vi "Calcu_STD Pressure_PB.vi"(6 "Resolution":string[][](array[string]), 9 "Dead Weight":string[][](array[string]), 10 "Cal STD":string[](array[string]), 11 "Condition":string[][](array[string])) -> (0 "배열":dbl[](array[numeric]), 1 "Mass set":string[][](array[string]), 2 "Uncertainty":string[][](array[string]), 3 "Data Out":string[][](array[string]), 4 "Weight set":string[][](array[string]), 5 "STD Data":string[][](array[string]))   [LabVIEW 2020]
uses:
  Controls/Cmd_File path.ctl
  Controls/Cmd_File Type.ctl
  Public/Polymorph/Data Class_2D Str.vi
  Variables/Global_Cal Info.vi
  Public/Polymorph/Array Dedup_2D Str.vi
  Public/Polymorph/Sort_2D Str.vi
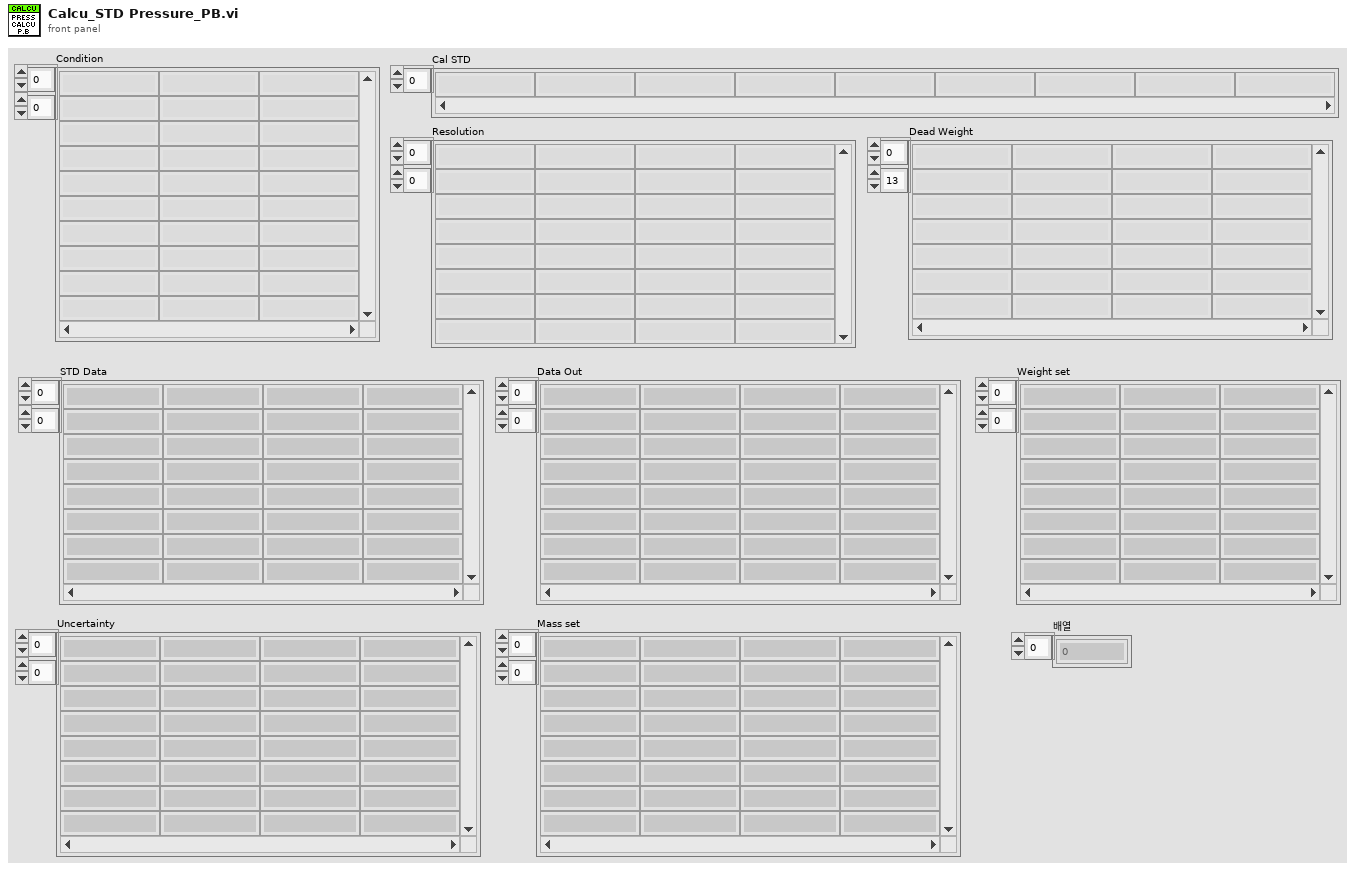
[diagram p1: front panel]
types:
  T1 = typedef "Cmd_File Type.ctl" = enum16{"엑셀", "엑셀(2003)", "텍스트", "설정", "2진", "VI", "CSV", "LOG", "폴더"}
  T2 = typedef "Cmd_File path.ctl" = enum16{"에러로그", "데이터파일경로", "성적서원본", "지난성적서", "Data Files", "경로생성", "Updater", "Template", "설정파일경로", "FTP Upload", "Update 경로", "어플리케이션"}
  T3 = cluster{"세부분류코드":string, "형식":string, "옵션":string, "측정기명":string, "EXCEL파일명":string, "TEMP":string}
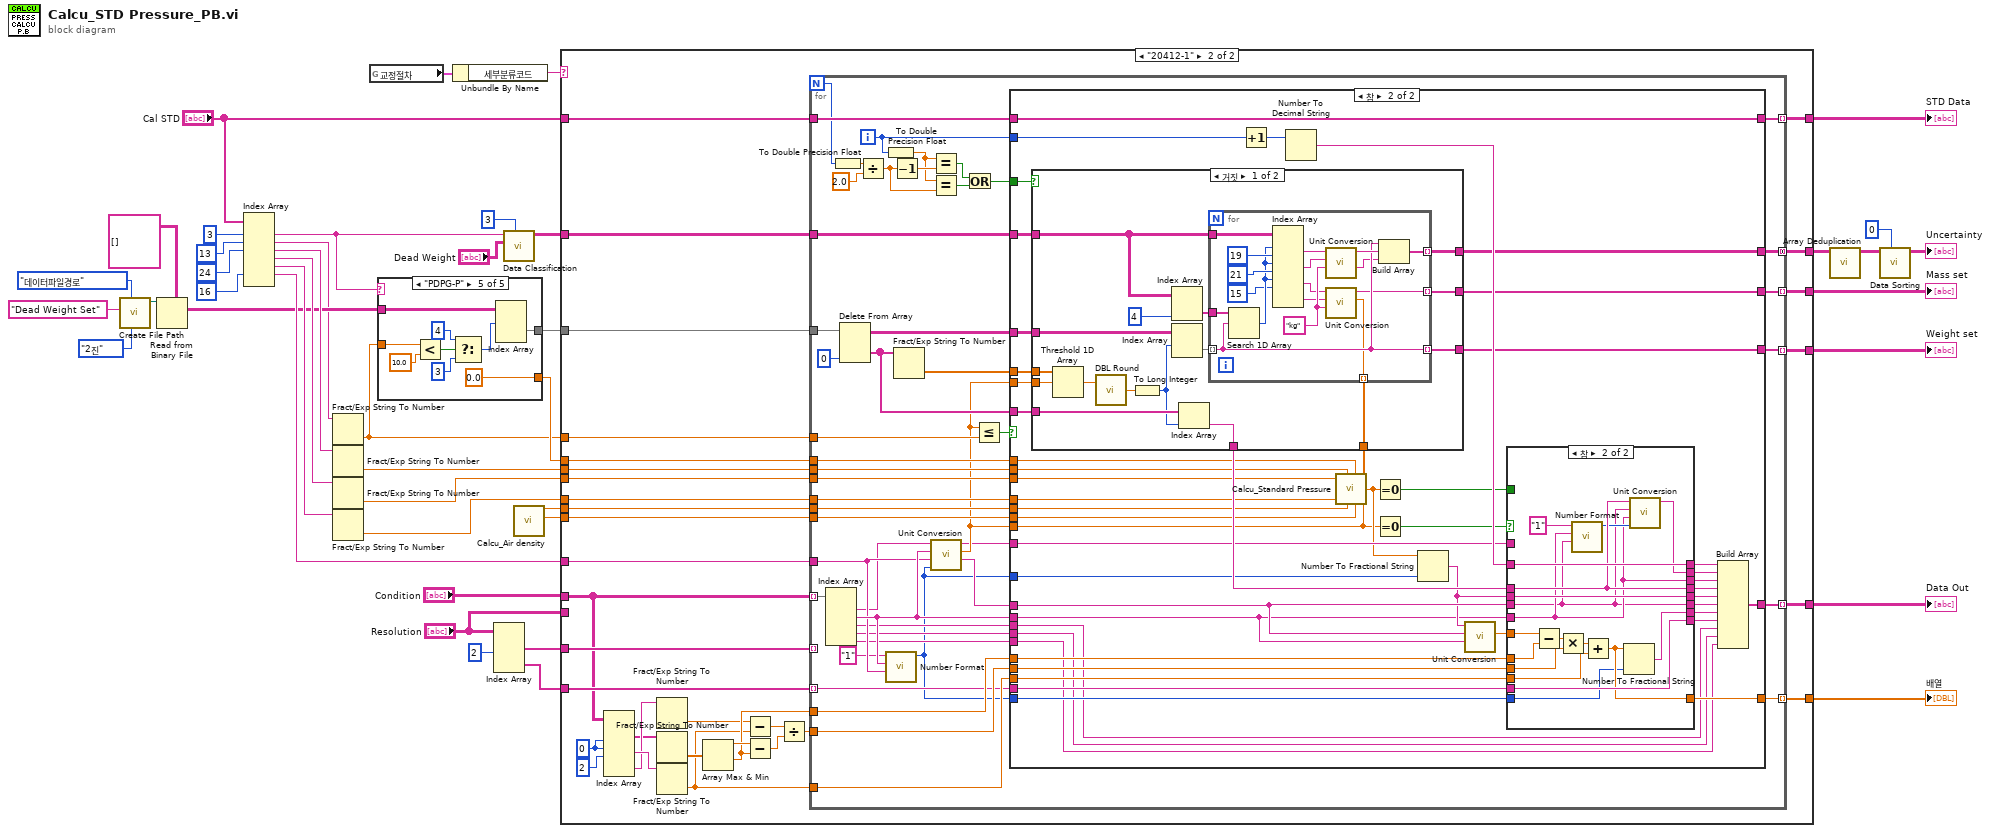
[diagram p0: block diagram]
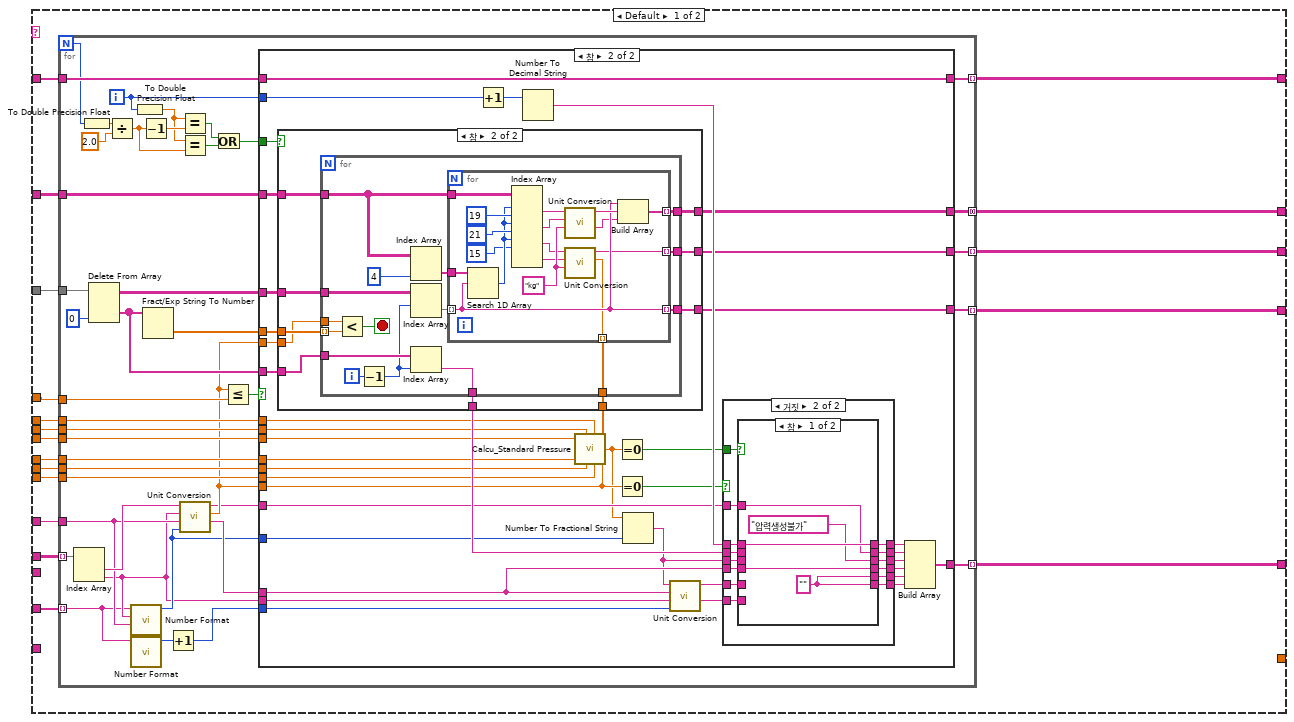
[diagram p2: hidden frame]
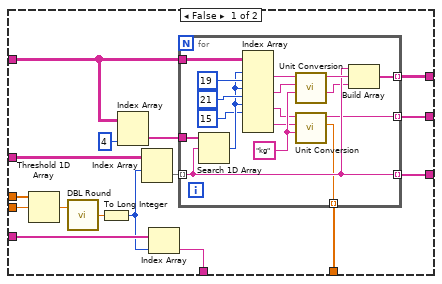
[diagram p6: hidden frame]
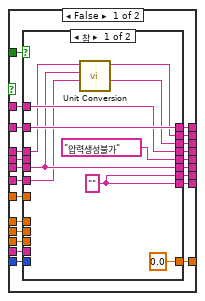
[diagram p8: hidden frame]
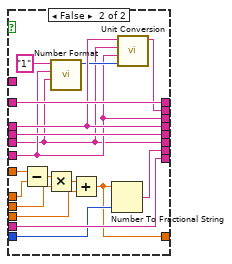
[diagram p9: hidden frame]
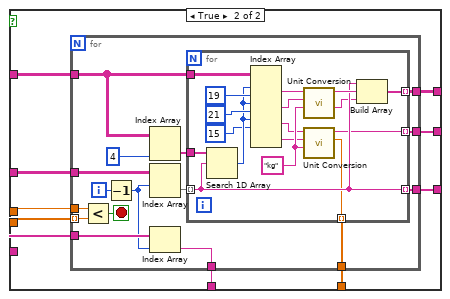
[diagram p10: hidden frame]
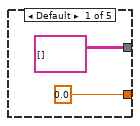
[diagram p11: hidden frame]
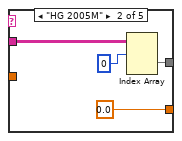
[diagram p12: hidden frame]
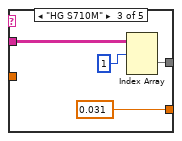
[diagram p13: hidden frame]
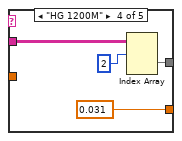
[diagram p14: hidden frame]
diagram:
  n1 = call "Create File Path.vi"("파일타입"=Cmd_File_Type."2진", "항목"=Cmd_File_path."데이터파일경로", "문자열 in"="Dead Weight Set") -> ("파일경로"=w7:path)  [unwired: 5 in, 3 out]
  n2 = Read from Binary File(5:string[][][] [], 11:w7) -> (2:w11:string[][][])  [unwired: 4 in, 3 out]
  n3 = Index Array(array="Cal STD", index #1=3 ("인덱스"), index #2=13 ("인덱스"), index #3=24 ("인덱스"), index #6=16 ("인덱스")) -> (element #1=w17:string, element #2=w6:string, element #3=w21:string, element #4=w20:string, element #5=w19:string, element #6=w14:string)  [unwired: 3 in, 1 out]
  n4 = Fract/Exp String To Number(string=w6) -> (number=w5:dbl)  [unwired: 3 in, 1 out]
  n5 = Fract/Exp String To Number(string=w21) -> (number=w35:dbl)  [unwired: 3 in, 1 out]
  n6 = Fract/Exp String To Number(string=w20) -> (number=w37:dbl)  [unwired: 3 in, 1 out]
  n7 = Fract/Exp String To Number(string=w19) -> (number=w36:dbl)  [unwired: 3 in, 1 out]
  n8 = global read "Global_Cal Info.vi" "교정절차"() -> (w24:T3)
  n9 = case shown="\"PDPG-P\"" w17 {
    tunnel: [string[][] [] ("테이블 컨트롤 2") w48 w51 w55 w65] -> w43
    tunnel: [0.0 0.0 0.031 0.031 0.0] -> w38
    tunnel: w11 -> [_ w49 w53 w57 w66]
    tunnel: w5 -> [_ _ _ _ w64]
    frame Default {
    }
    frame "HG 2005M" {
      n10 = Index Array(array=w49, index (dim 0)=0 ("인덱스 (페이지)")) -> (element=w48:string[][])  [unwired: 2 in]
    }
    frame "HG S710M" {
      n11 = Index Array(array=w53, index (dim 0)=1 ("인덱스 (페이지)")) -> (element=w51:string[][])  [unwired: 2 in]
    }
    frame "HG 1200M" {
      n12 = Index Array(array=w57, index (dim 0)=2 ("인덱스 (페이지)")) -> (element=w55:string[][])  [unwired: 2 in]
    }
    frame "PDPG-P" {
      n13 = Less?(x=w64, y=10.0) -> (x < y?=w62:bool)
      n14 = Select(t=4 ("인덱스 (페이지)"), s=w62, f=3 ("인덱스 (페이지)")) -> (s? t:f=w60:i32)
      n15 = Index Array(array=w66, index (dim 0)=w60) -> (element=w65:string[][])  [unwired: 2 in]
    }
  }
  n16 = Unbundle By Name(w24) -> ("세부분류코드"=w2:string)
  n17 = Index Array(array="Resolution", index (col) #1=2 ("비활성화된 인덱스 (열)")) -> (element #1=w33:string[], element #2=w23:string[])  [unwired: 3 in]
  n18 = call-poly "Data Classification.vi"("인덱스"=3, "DATA 입력"="Dead Weight", "검색 문자열"=w17) -> ("DATA 출력"=w40:string[][])  [unwired: 4 in, 4 out]
  n19 = call "Calcu_Air density.vi"() -> ("t(℃)"=w4:dbl, "ρ_air"=w39:dbl)  [unwired: 10 in]
  n20 = case shown="\"20412-1\"" w2 {
    tunnel: [w85 w306] -> w44
    tunnel: "Condition" -> [w84 w278]
    tunnel: w14 -> [w83 w305]
    tunnel: w43 -> [w82 w304]
    tunnel: w40 -> [w81 w303]
    tunnel: w39 -> [w80 w302]
    tunnel: w38 -> [w79 w301]
    tunnel: w37 -> [w78 w300]
    tunnel: w4 -> [w77 w299]
    tunnel: w36 -> [w76 w298]
    tunnel: w35 -> [w75 w297]
    tunnel: w5 -> [w74 w296]
    tunnel: w33 -> [w73 w295]
    tunnel: [w72 w294] -> w32
    tunnel: "Cal STD" -> [w71 w293]
    tunnel: [w70 w292] -> w27
    tunnel: [w69 w291] -> w26
    tunnel: [w68 w290] -> w25
    tunnel: w23 -> [_ w289]
    tunnel: [_ w288] -> w13
    tunnel: "Resolution" -> [_ _]
    frame Default {
      n21 = for {
        N -> [w101]
        tunnel: [w126] -> w85 mode=indexing
        tunnel: w84 -> [w125] mode=indexing
        tunnel: w83 -> [w104]
        tunnel: w82 -> [w122]
        tunnel: [w118] -> w69 mode=indexing
        tunnel: w81 -> [w121]
        tunnel: w80 -> [w117]
        tunnel: w79 -> [w116]
        tunnel: w75 -> [w115]
        tunnel: w78 -> [w114]
        tunnel: w77 -> [w113]
        tunnel: w76 -> [w112]
        tunnel: w74 -> [w110]
        tunnel: w73 -> [w88] mode=indexing
        tunnel: [w108] -> w72 mode=concatenating
        tunnel: w71 -> [w107]
        tunnel: [w106] -> w70 mode=indexing
        tunnel: [w105] -> w68 mode=indexing
        i -> [w97]
        n22 = Index Array(array=w125) -> (element #1=w124:string, element #2=w89:string)  [unwired: 2 in]
        n23 = To Double Precision Float(number=w101) -> (double precision float=w95:dbl)
        n24 = Delete From Array(array=w122, index (col)=0 ("비활성화된 인덱스 (열)")) -> (deleted portion=w103:string[], array with subset deleted=w119:string[][])  [unwired: 2 in]
        n25 = Divide(x=w95, y=2.0) -> (x/y=w99:dbl)
        n26 = call "Number Format.vi"("기준단위"=w104, "입력단위"=w89, "입력값"=w88) -> ("정밀도(단위적용)"=w91:i32)  [unwired: 8 in]
        n27 = call "Number Format.vi"("입력값"=w88) -> ("정밀도(단위적용)"=w87:i32)  [unwired: 10 in]
        n28 = To Double Precision Float(number=w97) -> (double precision float=w96:dbl)
        n29 = Decrement(x=w99) -> (x-1=w98:dbl)
        n30 = Fract/Exp String To Number(string=w103) -> (number=w123:dbl[])  [unwired: 3 in, 1 out]
        n31 = Increment(x=w87) -> (x+1=w86:i32)
        n32 = Equal?(x=w96, y=w98) -> (x = y?=w94:bool)
        n33 = Equal?(x=w96, y=w99) -> (x = y?=w93:bool)
        n34 = call "Unit Conversion.vi"("소수점 자리수"=w91, "환산단위"=w104, "입력단위"=w89, "입력값"=w124) -> ("환산단위"=w111:string, "환산값 (DBL)"=w102:dbl, "환산값 (string)"=w92:string)  [unwired: 2 in, 3 out]
        n35 = Or(x=w94, y=w93) -> (x .or. y?=w90:bool)
        n36 = Less Or Equal?(x=w102, y=w110) -> (x <= y?=w109:bool)
        n37 = case shown="참" w109 {
          tunnel: w97 -> [_ w166]
          tunnel: [_ w145] -> w126
          tunnel: w123 -> [_ w158]
          tunnel: w121 -> [_ w163]
          tunnel: w119 -> [_ w156]
          tunnel: [_ w137] -> w118
          tunnel: w117 -> [_ w130]
          tunnel: w116 -> [_ w134]
          tunnel: w115 -> [_ w133]
          tunnel: w114 -> [_ w132]
          tunnel: w102 -> [_ w157]
          tunnel: w113 -> [_ w129]
          tunnel: w112 -> [_ w131]
          tunnel: w111 -> [_ w149]
          tunnel: w89 -> [_ w150]
          tunnel: [_ w162] -> w108
          tunnel: w107 -> [_ w161]
          tunnel: [_ w161] -> w106
          tunnel: [_ w138] -> w105
          tunnel: w91 -> [_ w152]
          tunnel: w103 -> [_ w160]
          tunnel: w102 -> [_ w128]
          tunnel: w90 -> [_ w155]
          tunnel: w92 -> [_ w153]
          tunnel: w86 -> [_ w136]
          frame False {
          }
          frame True {
            n38 = case shown="참" w155 {
              tunnel: w163 -> [w209 w240]
              tunnel: [w206 w239] -> w137
              tunnel: [w207 w238] -> w162
              tunnel: [w204 w237] -> w135
              tunnel: [w205 w236] -> w138
              tunnel: w160 -> [w211 w235]
              tunnel: [w208 w234] -> w159
              tunnel: w158 -> [w202 w233]
              tunnel: w157 -> [w201 w232]
              tunnel: w156 -> [w210 w231]
              frame False {
                n39 = Threshold 1D Array(2:w201, 3:w202) -> (0:w198:dbl)  [unwired: 1 in]
                n40 = call "DBL Round.vi"("DBL in"=w198) -> ("DBL out"=w199:dbl)  [unwired: 2 in]
                n41 = To Long Integer(number=w199) -> (32bit integer=w203:i32)
                n42 = Index Array(array=w209, index (col)=4 ("비활성화된 인덱스 (열)")) -> (element=w213:string[])  [unwired: 1 in]
                n43 = Index Array(array=w210, index (row)=w203) -> (element=w212:string[])  [unwired: 1 in]
                n44 = Index Array(array=w211, index=w203) -> (element=w208:string)
                n45 = for {
                  tunnel: w212 -> [w223] mode=indexing
                  tunnel: w209 -> [w230]
                  tunnel: [w221] -> w206 mode=indexing
                  tunnel: [w224] -> w207 mode=indexing
                  tunnel: [w220] -> w204 mode=indexing
                  tunnel: [w223] -> w205 mode=indexing
                  tunnel: w213 -> [w219]
                  w222 = "kg" ("환산단위")
                  n46 = Search 1D Array(1D array=w219, element=w223) -> (index of element=w217:i32)  [unwired: 1 in]
                  n47 = Index Array(array=w230, index (row) #1=w217, index (col) #1=19 ("인덱스 (열)"), index (row) #2=w217, index (col) #2=21 ("인덱스 (열)"), index (row) #3=w217, index (col) #3=15 ("비활성화된 인덱스 (열)")) -> (element #1=w227:string, element #2=w226:string, element #3=w215:string, element #4=w214:string)  [unwired: 2 in]
                  n48 = call "Unit Conversion.vi"("환산단위"=w222, "입력단위"=w226, "입력값"=w227) -> ("환산단위"=w218:string, "환산값 (string)"=w225:string)  [unwired: 3 in, 4 out]
                  n49 = call "Unit Conversion.vi"("환산단위"=w222, "입력단위"=w214, "입력값"=w215) -> ("환산값 (DBL)"=w220:dbl, "환산값 (string)"=w221:string)  [unwired: 3 in, 4 out]
                  n50 = Build Array(w223, w225, w218) -> (w224:string[])
                }
              }
              frame True {
                n51 = for {
                  tunnel: w232 -> [w255]
                  tunnel: w233 -> [w256] mode=indexing
                  tunnel: w231 -> [w253]
                  tunnel: [w250] -> w239
                  tunnel: w240 -> [w242]
                  tunnel: [w249] -> w238
                  tunnel: [w248] -> w237
                  tunnel: [w247] -> w236
                  tunnel: w235 -> [w246]
                  tunnel: [w244] -> w234
                  i -> [w252]
                  stop <- w254 stop-if-true
                  n52 = Less?(x=w255, y=w256) -> (x < y?=w254:bool)
                  n53 = Decrement(x=w252) -> (x-1=w245:i32)
                  n54 = Index Array(array=w242, index (col)=4 ("비활성화된 인덱스 (열)")) -> (element=w241:string[])  [unwired: 1 in]
                  n55 = Index Array(array=w253, index (row)=w245) -> (element=w251:string[])  [unwired: 1 in]
                  n56 = Index Array(array=w246, index=w245) -> (element=w244:string)
                  n57 = for {
                    tunnel: w251 -> [w266] mode=indexing
                    tunnel: w242 -> [w273]
                    tunnel: [w264] -> w250 mode=indexing
                    tunnel: [w267] -> w249 mode=indexing
                    tunnel: [w263] -> w248 mode=indexing
                    tunnel: [w266] -> w247 mode=indexing
                    tunnel: w241 -> [w262]
                    w265 = "kg" ("환산단위")
                    n58 = Search 1D Array(1D array=w262, element=w266) -> (index of element=w260:i32)  [unwired: 1 in]
                    n59 = Index Array(array=w273, index (row) #1=w260, index (col) #1=19 ("인덱스 (열)"), index (row) #2=w260, index (col) #2=21 ("인덱스 (열)"), index (row) #3=w260, index (col) #3=15 ("비활성화된 인덱스 (열)")) -> (element #1=w270:string, element #2=w269:string, element #3=w258:string, element #4=w257:string)  [unwired: 2 in]
                    n60 = call "Unit Conversion.vi"("환산단위"=w265, "입력단위"=w269, "입력값"=w270) -> ("환산단위"=w261:string, "환산값 (string)"=w268:string)  [unwired: 3 in, 4 out]
                    n61 = call "Unit Conversion.vi"("환산단위"=w265, "입력단위"=w257, "입력값"=w258) -> ("환산값 (DBL)"=w263:dbl, "환산값 (string)"=w264:string)  [unwired: 3 in, 4 out]
                    n62 = Build Array(w266, w268, w261) -> (w267:string[])
                  }
                }
              }
            }
            n63 = Increment(x=w166) -> (x+1=w165:i32)
            n64 = Number To Decimal String(number=w165) -> (decimal integer string=w164:string)  [unwired: 1 in]
            n65 = call "Calcu_Standard Pressure.vi"("λ"=w132, "A0"=w133, "Ts"=w131, "ρa"=w130, "σ"=w134, "M"=w135, "Ta"=w129, "P"=w128) -> ("결과"=w127:dbl)  [unwired: 1 in]
            n66 = Equal To 0?(x=w127) -> (x = 0?=w151:bool)
            n67 = Equal To 0?(x=w128) -> (x = 0?=w154:bool)
            n68 = Number To Fractional String(number=w127, precision (6)=w152) -> (F-format string=w148:string)  [unwired: 2 in]
            n69 = call "Unit Conversion.vi"("소수점 자리수"=w136, "환산단위"=w150, "입력단위"=w149, "입력값"=w148) -> ("환산단위"=w146:string, "환산값 (string)"=w147:string)  [unwired: 2 in, 4 out]
            n70 = case shown="거짓" w154 {
              tunnel: w164 -> [w172 w186]
              tunnel: w149 -> [w169 w185]
              tunnel: w159 -> [w171 w184]
              tunnel: w153 -> [_ w183]
              tunnel: w148 -> [w170 w182]
              tunnel: w151 -> [_ w181]
              tunnel: w147 -> [w168 w179]
              tunnel: w146 -> [w167 w180]
              tunnel: [w172 w178] -> w144
              tunnel: [w171 w177] -> w143
              tunnel: [w170 w176] -> w142
              tunnel: [w169 w175] -> w141
              tunnel: [w168 w174] -> w140
              tunnel: [w167 w173] -> w139
              frame True {
              }
              frame False {
                n71 = case shown="참" w181 {
                  tunnel: w186 -> [w191 w197]
                  tunnel: w185 -> [w188 w194]
                  tunnel: w184 -> [_ w196]
                  tunnel: w183 -> [w190 _]
                  tunnel: w182 -> [_ w195]
                  tunnel: w180 -> [_ w192]
                  tunnel: w179 -> [_ w193]
                  tunnel: [w191 w197] -> w178
                  tunnel: [w190 w196] -> w177
                  tunnel: ["압력생성불가" w195] -> w176
                  tunnel: [w188 w194] -> w175
                  tunnel: [w187 w193] -> w174
                  tunnel: [w187 w192] -> w173
                  frame True {
                    w187 = ""
                  }
                  frame False {
                  }
                }
              }
            }
            n72 = Build Array(w144, w143, w142, w141, w140, w139) -> (w145:string[])
          }
        }
      }
    }
    frame "20412-1" {
      w275 = 0 ("비활성화된 인덱스 (열)")
      n73 = Index Array(array=w278, index (col) #1=w275, index (row) #2=w275, index (col) #2=2 ("인덱스 (행)")) -> (element #1=w274:string[], element #2=w277:string, element #3=w276:string)  [unwired: 3 in]
      n74 = Fract/Exp String To Number(string=w276) -> (number=w281:dbl)  [unwired: 3 in, 1 out]
      n75 = Fract/Exp String To Number(string=w274) -> (number=w282:dbl[])  [unwired: 3 in, 1 out]
      n76 = Fract/Exp String To Number(string=w277) -> (number=w280:dbl)  [unwired: 3 in, 1 out]
      n77 = Array Max & Min(array=w282) -> (max value=w284:dbl, min value=w283:dbl)  [unwired: 2 out]
      n78 = Subtract(x=w281, y=w280) -> (x-y=w286:dbl)
      n79 = Subtract(x=w284, y=w283) -> (x-y=w285:dbl)
      n80 = Divide(x=w286, y=w285) -> (x/y=w287:dbl)
      n81 = for {
        N -> [w328]
        tunnel: [w353] -> w306 mode=indexing
        tunnel: w278 -> [w352] mode=indexing
        tunnel: w305 -> [w331]
        tunnel: w304 -> [w350]
        tunnel: [w346] -> w291 mode=indexing
        tunnel: w303 -> [w349]
        tunnel: w302 -> [w345]
        tunnel: w301 -> [w344]
        tunnel: w297 -> [w343]
        tunnel: w300 -> [w342]
        tunnel: w299 -> [w341]
        tunnel: w298 -> [w340]
        tunnel: w296 -> [w338]
        tunnel: w295 -> [_] mode=indexing
        tunnel: [w336] -> w294 mode=concatenating
        tunnel: w293 -> [w335]
        tunnel: [w334] -> w292 mode=indexing
        tunnel: [w333] -> w290 mode=indexing
        tunnel: w287 -> [w317]
        tunnel: w283 -> [w316]
        tunnel: w280 -> [w315]
        tunnel: w289 -> [w314] mode=indexing
        tunnel: [w313] -> w288 mode=indexing
        i -> [w324]
        n82 = Index Array(array=w352) -> (element #1=w308:string, element #2=w332:string, element #3=w312:string, element #4=w311:string, element #5=w310:string)  [unwired: 5 in]
        n83 = To Double Precision Float(number=w328) -> (double precision float=w322:dbl)
        n84 = Delete From Array(array=w350, index (col)=0 ("비활성화된 인덱스 (열)")) -> (deleted portion=w330:string[], array with subset deleted=w347:string[][])  [unwired: 2 in]
        n85 = Divide(x=w322, y=2.0) -> (x/y=w326:dbl)
        n86 = To Double Precision Float(number=w324) -> (double precision float=w323:dbl)
        n87 = call "Number Format.vi"("기준단위"=w331, "입력단위"=w332, "입력값"="1") -> ("정밀도(단위적용)"=w309:i32)  [unwired: 8 in]
        n88 = Decrement(x=w326) -> (x-1=w325:dbl)
        n89 = Fract/Exp String To Number(string=w330) -> (number=w351:dbl[])  [unwired: 3 in, 1 out]
        n90 = Equal?(x=w323, y=w325) -> (x = y?=w321:bool)
        n91 = Equal?(x=w323, y=w326) -> (x = y?=w320:bool)
        n92 = call "Unit Conversion.vi"("소수점 자리수"=w309, "환산단위"=w331, "입력단위"=w332, "입력값"=w308) -> ("환산단위"=w339:string, "환산값 (DBL)"=w329:dbl, "환산값 (string)"=w318:string)  [unwired: 2 in, 3 out]
        n93 = Or(x=w321, y=w320) -> (x .or. y?=w319:bool)
        n94 = Less Or Equal?(x=w329, y=w338) -> (x <= y?=w337:bool)
        n95 = case shown="참" w337 {
          tunnel: w324 -> [_ w402]
          tunnel: [_ w382] -> w353
          tunnel: w351 -> [_ w392]
          tunnel: w349 -> [_ w399]
          tunnel: w347 -> [_ w390]
          tunnel: [_ w398] -> w346
          tunnel: w345 -> [_ w355]
          tunnel: w344 -> [_ w360]
          tunnel: w343 -> [_ w359]
          tunnel: w342 -> [_ w358]
          tunnel: w329 -> [_ w391]
          tunnel: w341 -> [_ w356]
          tunnel: w340 -> [_ w354]
          tunnel: w339 -> [_ w384]
          tunnel: w332 -> [_ w365]
          tunnel: [_ w397] -> w336
          tunnel: w335 -> [_ w396]
          tunnel: [_ w396] -> w334
          tunnel: [_ w395] -> w333
          tunnel: w309 -> [_ w386]
          tunnel: w309 -> [_ w370]
          tunnel: w330 -> [_ w394]
          tunnel: w329 -> [_ w357]
          tunnel: w319 -> [_ w389]
          tunnel: w318 -> [_ w387]
          tunnel: w317 -> [_ w373]
          tunnel: w316 -> [_ w374]
          tunnel: w315 -> [_ w372]
          tunnel: w314 -> [_ w371]
          tunnel: [_ w369] -> w313
          tunnel: w312 -> [_ w368]
          tunnel: w311 -> [_ w367]
          tunnel: w310 -> [_ w366]
          frame False {
          }
          frame True {
            n96 = case shown="거짓" w389 {
              tunnel: w399 -> [w482 w513]
              tunnel: [w479 w512] -> w398
              tunnel: [w480 w511] -> w397
              tunnel: [w477 w510] -> w361
              tunnel: [w478 w509] -> w395
              tunnel: w394 -> [w484 w508]
              tunnel: [w481 w507] -> w393
              tunnel: w392 -> [w475 w506]
              tunnel: w391 -> [w474 w505]
              tunnel: w390 -> [w483 w504]
              frame False {
                n97 = Threshold 1D Array(2:w474, 3:w475) -> (0:w471:dbl)  [unwired: 1 in]
                n98 = call "DBL Round.vi"("DBL in"=w471) -> ("DBL out"=w472:dbl)  [unwired: 2 in]
                n99 = To Long Integer(number=w472) -> (32bit integer=w476:i32)
                n100 = Index Array(array=w482, index (col)=4 ("비활성화된 인덱스 (열)")) -> (element=w486:string[])  [unwired: 1 in]
                n101 = Index Array(array=w483, index (row)=w476) -> (element=w485:string[])  [unwired: 1 in]
                n102 = Index Array(array=w484, index=w476) -> (element=w481:string)
                n103 = for {
                  tunnel: w485 -> [w496] mode=indexing
                  tunnel: w482 -> [w503]
                  tunnel: [w494] -> w479 mode=indexing
                  tunnel: [w497] -> w480 mode=indexing
                  tunnel: [w493] -> w477 mode=indexing
                  tunnel: [w496] -> w478 mode=indexing
                  tunnel: w486 -> [w492]
                  w495 = "kg" ("환산단위")
                  n104 = Search 1D Array(1D array=w492, element=w496) -> (index of element=w490:i32)  [unwired: 1 in]
                  n105 = Index Array(array=w503, index (row) #1=w490, index (col) #1=19 ("인덱스 (열)"), index (row) #2=w490, index (col) #2=21 ("인덱스 (열)"), index (row) #3=w490, index (col) #3=15 ("비활성화된 인덱스 (열)")) -> (element #1=w500:string, element #2=w499:string, element #3=w488:string, element #4=w487:string)  [unwired: 2 in]
                  n106 = call "Unit Conversion.vi"("환산단위"=w495, "입력단위"=w499, "입력값"=w500) -> ("환산단위"=w491:string, "환산값 (string)"=w498:string)  [unwired: 3 in, 4 out]
                  n107 = call "Unit Conversion.vi"("환산단위"=w495, "입력단위"=w487, "입력값"=w488) -> ("환산값 (DBL)"=w493:dbl, "환산값 (string)"=w494:string)  [unwired: 3 in, 4 out]
                  n108 = Build Array(w496, w498, w491) -> (w497:string[])
                }
              }
              frame True {
                n109 = for {
                  tunnel: w505 -> [w528]
                  tunnel: w506 -> [w529] mode=indexing
                  tunnel: w504 -> [w526]
                  tunnel: [w523] -> w512
                  tunnel: w513 -> [w515]
                  tunnel: [w522] -> w511
                  tunnel: [w521] -> w510
                  tunnel: [w520] -> w509
                  tunnel: w508 -> [w519]
                  tunnel: [w517] -> w507
                  i -> [w525]
                  stop <- w527 stop-if-true
                  n110 = Less?(x=w528, y=w529) -> (x < y?=w527:bool)
                  n111 = Decrement(x=w525) -> (x-1=w518:i32)
                  n112 = Index Array(array=w515, index (col)=4 ("비활성화된 인덱스 (열)")) -> (element=w514:string[])  [unwired: 1 in]
                  n113 = Index Array(array=w526, index (row)=w518) -> (element=w524:string[])  [unwired: 1 in]
                  n114 = Index Array(array=w519, index=w518) -> (element=w517:string)
                  n115 = for {
                    tunnel: w524 -> [w539] mode=indexing
                    tunnel: w515 -> [w546]
                    tunnel: [w537] -> w523 mode=indexing
                    tunnel: [w540] -> w522 mode=indexing
                    tunnel: [w536] -> w521 mode=indexing
                    tunnel: [w539] -> w520 mode=indexing
                    tunnel: w514 -> [w535]
                    w538 = "kg" ("환산단위")
                    n116 = Search 1D Array(1D array=w535, element=w539) -> (index of element=w533:i32)  [unwired: 1 in]
                    n117 = Index Array(array=w546, index (row) #1=w533, index (col) #1=19 ("인덱스 (열)"), index (row) #2=w533, index (col) #2=21 ("인덱스 (열)"), index (row) #3=w533, index (col) #3=15 ("비활성화된 인덱스 (열)")) -> (element #1=w543:string, element #2=w542:string, element #3=w531:string, element #4=w530:string)  [unwired: 2 in]
                    n118 = call "Unit Conversion.vi"("환산단위"=w538, "입력단위"=w542, "입력값"=w543) -> ("환산단위"=w534:string, "환산값 (string)"=w541:string)  [unwired: 3 in, 4 out]
                    n119 = call "Unit Conversion.vi"("환산단위"=w538, "입력단위"=w530, "입력값"=w531) -> ("환산값 (DBL)"=w536:dbl, "환산값 (string)"=w537:string)  [unwired: 3 in, 4 out]
                    n120 = Build Array(w539, w541, w534) -> (w540:string[])
                  }
                }
              }
            }
            n121 = Increment(x=w402) -> (x+1=w401:i32)
            n122 = Number To Decimal String(number=w401) -> (decimal integer string=w400:string)  [unwired: 1 in]
            n123 = call "Calcu_Standard Pressure.vi"("λ"=w358, "A0"=w359, "Ts"=w354, "ρa"=w355, "σ"=w360, "M"=w361, "Ta"=w356, "P"=w357) -> ("결과"=w362:dbl)  [unwired: 1 in]
            n124 = Equal To 0?(x=w362) -> (x = 0?=w385:bool)
            n125 = Equal To 0?(x=w357) -> (x = 0?=w388:bool)
            n126 = Number To Fractional String(number=w362, precision (6)=w386) -> (F-format string=w383:string)  [unwired: 2 in]
            n127 = call "Unit Conversion.vi"("환산단위"=w365, "입력단위"=w384, "입력값"=w383) -> ("환산값 (DBL)"=w375:dbl)  [unwired: 3 in, 5 out]
            n128 = case shown="참" w388 {
              tunnel: w400 -> [w424 w470]
              tunnel: w384 -> [w423 w453]
              tunnel: w393 -> [w422 w458]
              tunnel: w387 -> [w421 _]
              tunnel: w383 -> [w420 w469]
              tunnel: w385 -> [w419 _]
              tunnel: [w418 w470] -> w381
              tunnel: [w417 w458] -> w380
              tunnel: [w416 w469] -> w379
              tunnel: [w415 w453] -> w378
              tunnel: [w414 w468] -> w377
              tunnel: [w413 w463] -> w376
              tunnel: w375 -> [w412 w467]
              tunnel: w374 -> [w411 w466]
              tunnel: w373 -> [w410 w465]
              tunnel: w372 -> [w409 w464]
              tunnel: w371 -> [w408 w463]
              tunnel: w370 -> [w407 w459]
              tunnel: [w406 w460] -> w369
              tunnel: w365 -> [w405 w454]
              tunnel: [w404 w457] -> w364
              tunnel: [w403 w454] -> w363
              frame False {
                n129 = case shown="참" w419 {
                  tunnel: w424 -> [w434 w452]
                  tunnel: w423 -> [w428 w435]
                  tunnel: w422 -> [w429 w440]
                  tunnel: w421 -> [w433 _]
                  tunnel: w420 -> [_ w451]
                  tunnel: [w434 w452] -> w418
                  tunnel: [w433 w440] -> w417
                  tunnel: ["압력생성불가" w451] -> w416
                  tunnel: [w428 w435] -> w415
                  tunnel: [w431 w444] -> w414
                  tunnel: [w431 w443] -> w413
                  tunnel: w412 -> [_ w448]
                  tunnel: w411 -> [_ w447]
                  tunnel: w410 -> [_ w446]
                  tunnel: w409 -> [_ w445]
                  tunnel: w408 -> [_ w443]
                  tunnel: w407 -> [_ w442]
                  tunnel: [0.0 w441] -> w406
                  tunnel: w405 -> [w427 w436]
                  tunnel: [w426 w439] -> w404
                  tunnel: [w425 w436] -> w403
                  frame True {
                    w431 = ""
                    n130 = call "Unit Conversion.vi"("환산단위"=w427, "입력단위"=w428, "입력값"=w429) -> ("환산단위"=w425:string, "환산값 (string)"=w426:string)  [unwired: 3 in, 4 out]
                  }
                  frame False {
                    n131 = Subtract(x=w448, y=w447) -> (x-y=w450:dbl)
                    n132 = Multiply(x=w450, y=w446) -> (x*y=w449:dbl)
                    n133 = call "Number Format.vi"("기준단위"=w435, "입력단위"=w436, "입력값"="1") -> ("정밀도(단위적용)"=w437:i32)  [unwired: 8 in]
                    n134 = Add(x=w449, y=w445) -> (x+y=w441:dbl)
                    n135 = Number To Fractional String(number=w441, precision (6)=w442) -> (F-format string=w444:string)  [unwired: 2 in]
                    n136 = call "Unit Conversion.vi"("소수점 자리수"=w437, "환산단위"=w436, "입력단위"=w435, "입력값"=w440) -> ("환산값 (string)"=w439:string)  [unwired: 2 in, 5 out]
                  }
                }
              }
              frame True {
                n137 = Subtract(x=w467, y=w466) -> (x-y=w462:dbl)
                n138 = Multiply(x=w462, y=w465) -> (x*y=w461:dbl)
                n139 = call "Number Format.vi"("기준단위"=w453, "입력단위"=w454, "입력값"="1") -> ("정밀도(단위적용)"=w456:i32)  [unwired: 8 in]
                n140 = Add(x=w461, y=w464) -> (x+y=w460:dbl)
                n141 = Number To Fractional String(number=w460, precision (6)=w459) -> (F-format string=w468:string)  [unwired: 2 in]
                n142 = call "Unit Conversion.vi"("소수점 자리수"=w456, "환산단위"=w454, "입력단위"=w453, "입력값"=w458) -> ("환산값 (string)"=w457:string)  [unwired: 2 in, 5 out]
              }
            }
            n143 = Build Array(w381, w364, w363, w380, w379, w378, w377, w376, w368, w367, w366) -> (w382:string[])
          }
        }
      }
    }
  }
  "Data Out" <- w44
  "STD Data" <- w27
  "Mass set" <- w26
  "Weight set" <- w25
  "배열" <- w13
  n144 = call-poly "Array Deduplication.vi"("배열 in"=w32) -> ("배열 out"=w31:string[][])  [unwired: 9 in, 1 out]
  n145 = call-poly "Data Sorting.vi"("기준열"=u16 0, "Data in"=w31) -> ("Data out"=→"Uncertainty":string[][])  [unwired: 8 in, 1 out]
